vi "Calibration Cold Limit (Read).vi"(6 "ISOBUS address":T3=-1 caption="ISOBUS address (-1)", 8 "error in":errorcluster, 11 "Mercury Reference In":T4) -> (0 "error out":errorcluster, 1 "Unit":T1, 2 "Cold Limit":dbl, 3 "Mercury Reference Out":T4, 4 "Valid?":T2)   [LabVIEW 2018, in "Mercury iXX.lvlib" / "Temperature.lvlib"]
doc: "Read the current cold limit of the selected temperature device."
uses:
  Temperature.lvlib
  Mercury Reference.ctl
  Comms Transport Layer.ctl
  Query Dynamic Reference.ctl
  ISOBus Address.ctl
  Is Valid LED.ctl
  Unit String.ctl
  Command Verbs.ctl
  Mercury iXX.lvlib
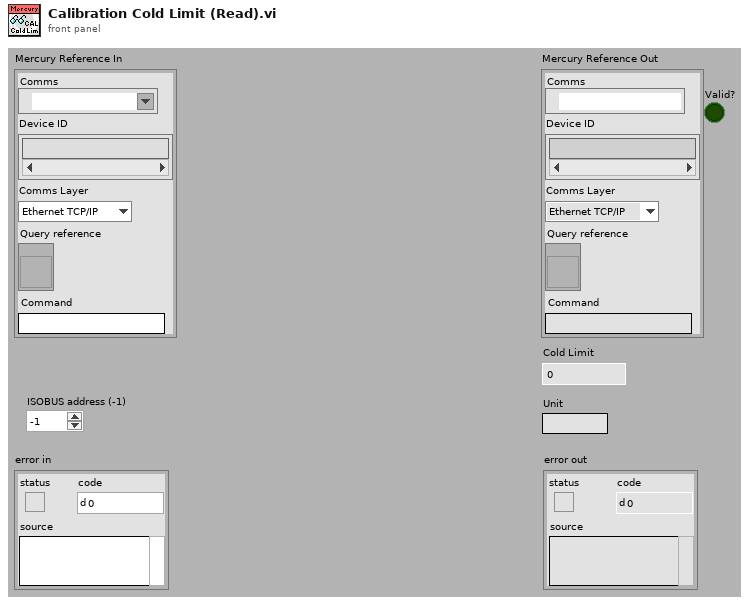
[diagram p1: front panel]
types:
  T1 = typedef "Mercury iXX.lvlib/Unit String.ctl" = string
  T2 = typedef "Mercury iXX.lvlib/Is Valid LED.ctl" = bool
  T3 = typedef "Mercury iXX.lvlib/ISOBus Address.ctl" = i32
  T4 = typedef "Mercury iXX.lvlib/Mercury Reference.ctl" = cluster{"Comms":refnum<visa-resource-name>, "Device ID":string[], "Comms Layer":T5, "Command":string, "Query reference":T6}
  T5 = typedef "Mercury iXX.lvlib/Comms Transport Layer.ctl" = enum16{"Ethernet TCP/IP", "USB", "ISOBus - RS-232", "GPIB"}
  T6 = typedef "Mercury iXX.lvlib/Query Dynamic Reference.ctl" = refnum<vi>
  T7 = typedef "Mercury iXX.lvlib/Command Verbs.ctl" = string
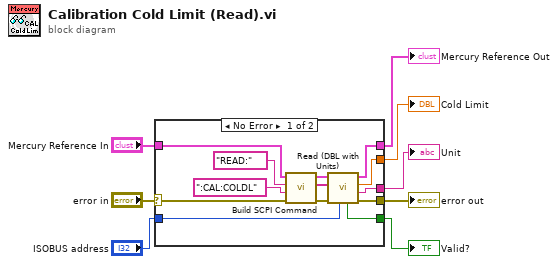
[diagram p0: block diagram]
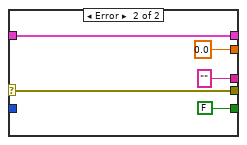
[diagram p2: hidden frame]
diagram:
  n1 = case shown="No Error" "error in" {
    selector: "error in" -> [w11 w26]
    tunnel: "Mercury Reference In" -> [w21 w25]
    tunnel: [w20 T1 "" ("Unit")] -> w7
    tunnel: [w19 0.0 ("Data (Dbl)")] -> w6
    tunnel: [w15 w25] -> w5
    tunnel: [w14 w26] -> w4
    tunnel: [w13 T2 FALSE ("Valid?")] -> w3
    tunnel: "ISOBUS address" -> [w12 _]
    frame No Error {
      n2 = call "Build SCPI Command.vi"("error in"=w11, "Noun(s)"=":CAL:COLDL" ("Command"), "Verb"=T7 "READ:", "Mercury Reference In"=w21) -> ("error out"=w18:errorcluster, "SCPI Message(s)"=w16:string[], "Mercury Reference Out"=w17:T4)  [unwired: 5 out]
      n3 = call "Read (DBL with Units).vi"("ISOBUS address"=w12, "error in"=w18, "SCPI Message(s)"=w16, "Mercury Reference In"=w17) -> ("error out"=w14:errorcluster, "Unit"=w20:T1, "Data (Dbl)"=w19:dbl, "Mercury Reference Out"=w15:T4, "Valid?"=w13:T2)  [unwired: 3 out]
    }
    frame Error {
    }
  }
  "Mercury Reference Out" <- w5
  "error out" <- w4
  "Cold Limit" <- w6
  "Valid?" <- w3
  "Unit" <- w7
